vi "Untitled 2.vi"() -> ()   [LabVIEW 2015, in "Copy of Untitled Library 1.lvlib"]
uses:
  Copy of Untitled Library 1.lvlib
  Controls/Enum Constant.ctl
  <userlib>/origin_lib_main/db_interface/DB Operations Enum.ctl
  <vilib>/addons/database/_DB Variant To Data/Database Variant To Data.xnode
  <userlib>/origin_lib_main/db_interface/DB Interface.lvlib
panel:
  out "Batch Open or Not":bool
  out "element":string
  in  "Cluster 2":cluster{"New":bool, "edit":bool, "Delete":bool}
  out "Cluster":cluster{"New":bool, "edit":bool, "Delete":bool}
  in  "Array":string[](array[string])
  out "error out":errorcluster
  in  "error in (no error) 5":errorcluster
  out "subarray":string[](array[string])
  out "format string":string
  in  "Module Number  2":dbl=1.0
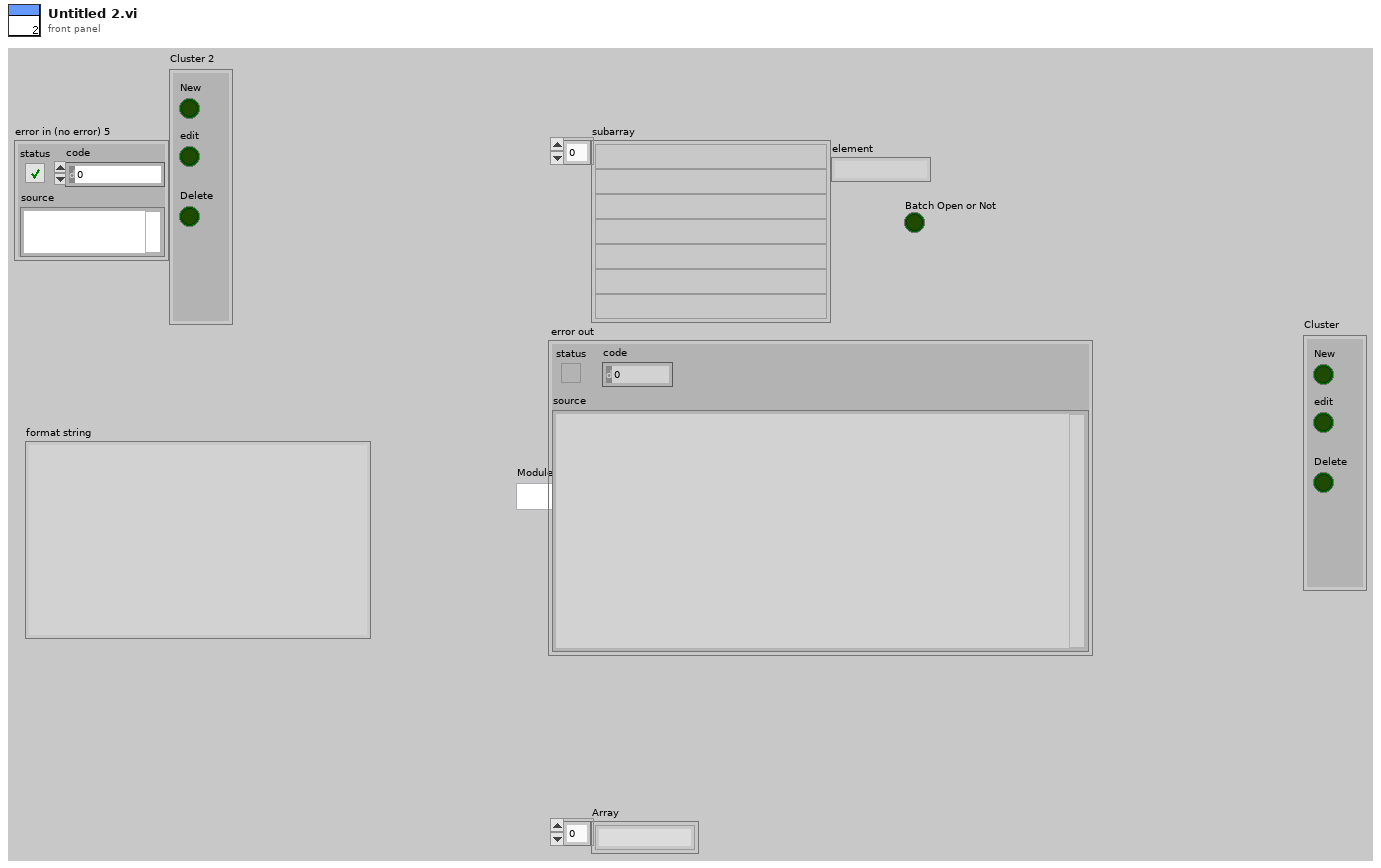
[diagram p1: front panel]
types:
  T1 = typedef "DB Interface.lvlib/DB Operations Enum.ctl" = enum16{"Select", "Update", "Insert", "Delete", "Fetch SQL Query", "Execute SQL Query", "Drop Table", "List Tables"}
  T2 = typedef "Enum Constant.ctl" = enum16{"Init", "Read", "Write"}
  T3 = typedef "FGV Data.ctl" = T4[]
  T4 = typedef "FGV Cluster Data.ctl" = cluster{"Manual/Automatic":bool, "UI Controllers ":string[], "UI Primery Key ":dbl[], "Caller Queue & MSG":T5, "Module ID":dbl, "DB Reference In":T6, "Products Columns":string[], "Cluster":cluster{"Delete Product":enum8{"Enabled", "Disabled", "Disabled and Grayed Out"}, "Add Product ":enum8{"Enabled", "Disabled", "Disabled and Grayed Out"}, "EDIT BATCH":enum8{"Enabled", "Disabled", "Disabled and Grayed Out"}, "Open Batch ":enum8{"Enabled", "Disabled", "Disabled and Grayed Out"}, "Close Batch":enum8{"Enabled", "Disabled", "Disabled and Grayed Out"}, "Delete Batch":enum8{"Enabled", "Disabled", "Disabled and Grayed Out"}, "Add Batch ":enum8{"Enabled", "Disabled", "Disabled and Grayed Out"}}}
  T5 = typedef "Queue and Caller MSG.ctl" = cluster{"Caller Queue":refnum<queue>, "Caller MSG":string}
  T6 = typedef "NI_Database_API.lvlib/Conn ObjectReference.ctl" = refnum<k1>
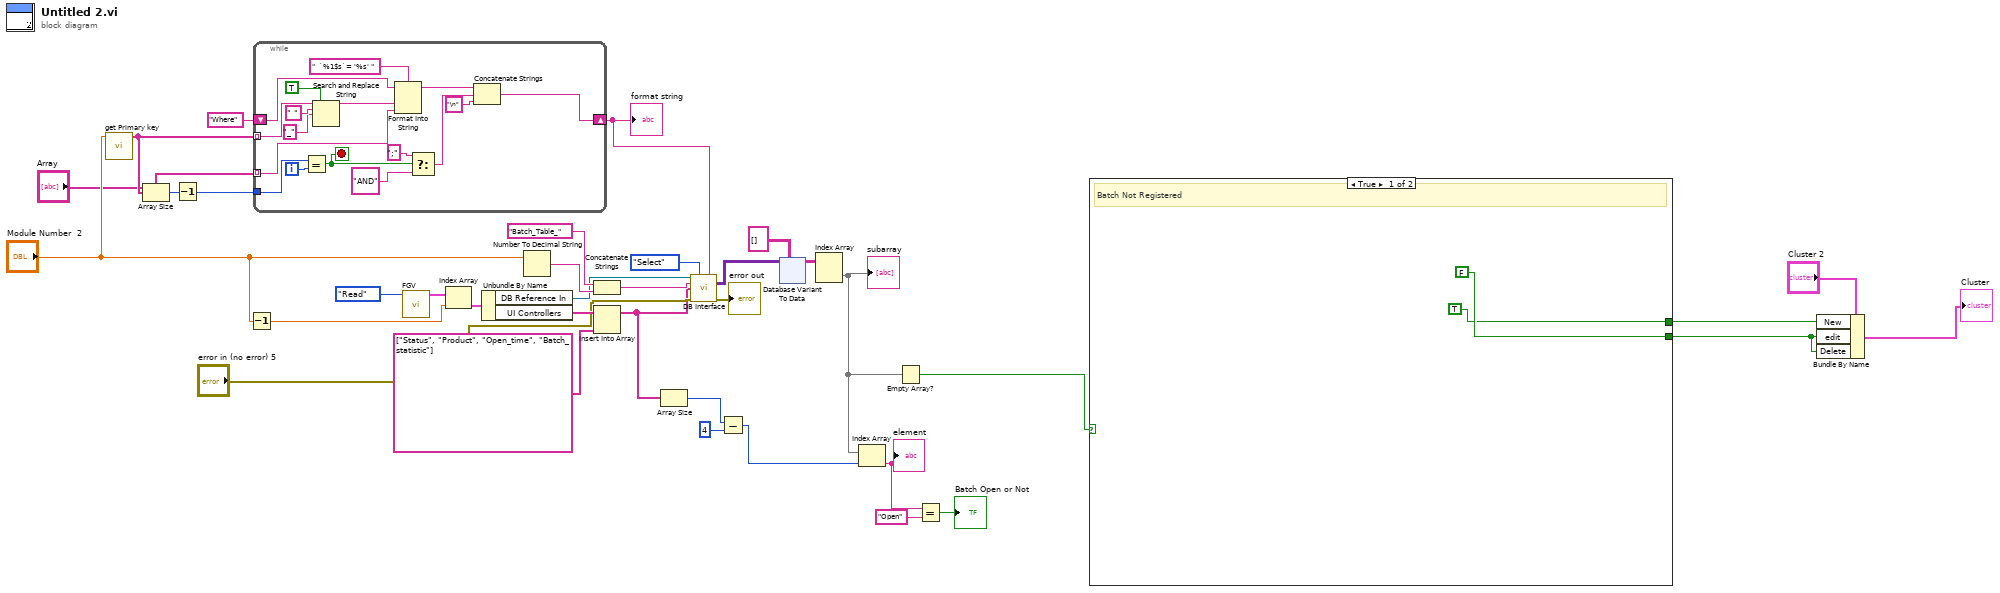
[diagram p0: block diagram]
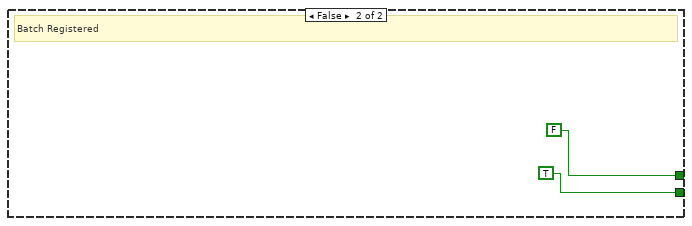
[diagram p2: hidden frame]
diagram:
  n1 = call "get Primary key.vi"("Module Number"="Module Number  2") -> ("Primery Key"=w18:string[])  [unwired: 10 in]
  n2 = Array Size(array=w18) -> (size(s)=w34:i32)
  n3 = Decrement(x=w34) -> (x-1=w33:i32)
  n4 = Decrement(x="Module Number  2") -> (x-1=w25:dbl)
  n5 = while {
    shift-right: [w40] -> w26
    shift-left: "Where" ("format string") -> [w52]
    tunnel: w33 -> [w46]
    tunnel: w18 -> [w41] mode=indexing
    tunnel: "Array" -> [w37] mode=indexing
    i -> [w47]
    stop <- w39 stop-if-true
    n6 = Equal?(x=w46, y=w47) -> (x = y?=w39:bool)
    n7 = Search and Replace String(replace all?=TRUE ("replace all? (F)"), input string=w41, search string=" ", replace string="_" ("replace string (\"\")")) -> (result string=w42:string)  [unwired: 4 in, 3 out]
    n8 = Format Into String(format string="  `%1$s`= '%s' ", initial string=w52, w42, w37) -> (resulting string=w51:string)  [unwired: 1 in, 1 out]
    n9 = Select(t=";", s=w39, f="AND") -> (s? t:f=w48:string)
    n10 = Concatenate Strings(w51, w48, "\n" ("string")) -> (w40:string)
  }
  "format string" <- w26
  n11 = call "FGV.vi"("Enum"=Enum_Constant."Read") -> ("Read Data"=w28:T3)  [unwired: 9 in, 1 out]
  n12 = Index Array(array=w28, index=w25) -> (element=w27:T4)
  n13 = Unbundle By Name(w27) -> ("DB Reference In"=w19:T6, "UI Controllers"=w16:string[])
  n14 = Number To Decimal String(number="Module Number  2") -> (decimal integer string=w30:string)  [unwired: 1 in]
  n15 = Concatenate Strings("Batch_Table_" ("string"), w30) -> (w29:string)
  n16 = Insert Into Array(array=w16, new element=string[] ["Status", "Product", "Open_time", "Batch_statistic"] ("element")) -> (w7:string[])  [unwired: 1 in]
  n17 = Array Size(array=w7) -> (size(s)=w6:i32)
  n18 = call <userlib>:"DB Interface.vi"("DB Ref In"=w19, "Operation"=DB_Operations_Enum."Select", "condition"=w26, "DB Table"=w29, "DB columns"=w7, "error in (no error)"="error in (no error) 5") -> ("data Out"=w21:variant[][], "error out"=→"error out":errorcluster)  [unwired: 6 in, 2 out]
  n19 = Subtract(x=w6, y=4) -> (x-y=w4:i32)
  n20 = xnode "Database Variant To Data"("database variant"=w21, "type"=string[][] [] ("columns")) -> ("data"=w22:string[][])  [unwired: 1 in, 1 out]
  n21 = Index Array(array=w22) -> (element=w8:string[])  [unwired: 2 in]
  "subarray" <- w8
  n22 = Index Array(array=w8, index=w4) -> (element=w3:string)
  "element" <- w3
  n23 = Empty Array?(array=w8) -> (empty?=w14:bool)
  n24 = Equal?(x=w3, y="Open") -> (x = y?=→"Batch Open or Not":bool)
  n25 = case shown="True" w14 {
    tunnel: [FALSE TRUE] -> w12
    tunnel: [TRUE FALSE] -> w11
    frame True {
      # "Batch Not Registered"
    }
    frame False {
      # "Batch Registered"
    }
  }
  n26 = Bundle By Name(cluster="Cluster 2", "New"=w11, "edit"=w12, "Delete"=w12) -> (→"Cluster":cluster{"New":bool, "edit":bool, "Delete":bool})
